vi "Convert Hex String to ASIIC.vi"(7 "Key? (T)":bool=TRUE, 9 "Hex":string) -> (1 "ASIIC":string)   [LabVIEW 2020, in "CBOR.lvlib"]
uses:
  CBOR.lvlib
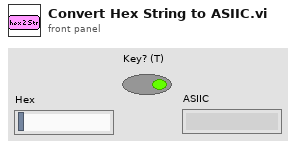
[diagram p1: front panel]
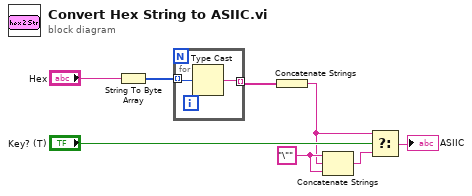
[diagram p0: block diagram]
diagram:
  w5 = "\"" ("string")
  n1 = String To Byte Array(string="Hex") -> (unsigned byte array=w3:u8[])
  n2 = for {
    tunnel: w3 -> [w10] mode=indexing
    tunnel: [w9] -> w2 mode=indexing
    n3 = Type Cast(x=w10) -> (*(type *) &x=w9:string)  [unwired: 1 in]
  }
  n4 = Concatenate Strings(w2) -> (w1:string)
  n5 = Concatenate Strings(w5, w1, w5) -> (w7:string)
  n6 = Select(t=w1, s="Key? (T)", f=w7) -> (s? t:f=→"ASIIC":string)
